vi "Configure Record Parameters (5772).vi"(6 "Record Count":u16=1, 7 "Record Length":u16=3000, 8 "error in":errorcluster, 9 "% of Acquisition Hold Off Time":dbl=10.0, 10 "% of Pre-Trigger Samples":dbl=10.0, 11 "FPGA VI Reference In":refnum<k20>) -> (0 "error out":errorcluster, 3 "FPGA VI Reference Out":refnum<k20>)   [LabVIEW 2012]
uses:
  <vilib>/rvi/errors/niLvFpgaAdjustHostInterfaceError.vi
  <vilib>/rvi/interface/nirviReadWriteControl/nirviReadWriteControl.xnode
  NiFpgaLv.dll
  <vilib>/rvi/interface/Simulation/niFpgaSimulationCallBeginRW.vi
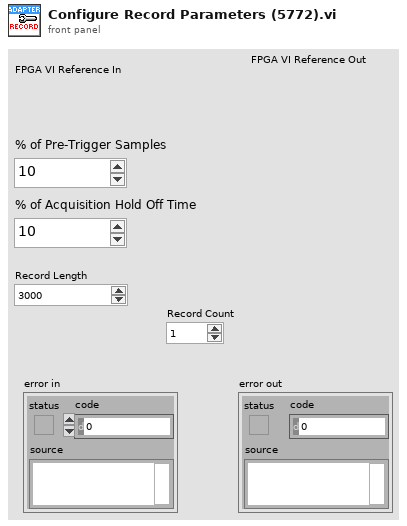
[diagram p1: front panel]
types:
  T1 = cluster{"Load Record Parameters?":bool, "Pre Trigger Samples":u16, "Samples per Record":u16, "Trigger Hold Off":u16, "Record Count":u16}
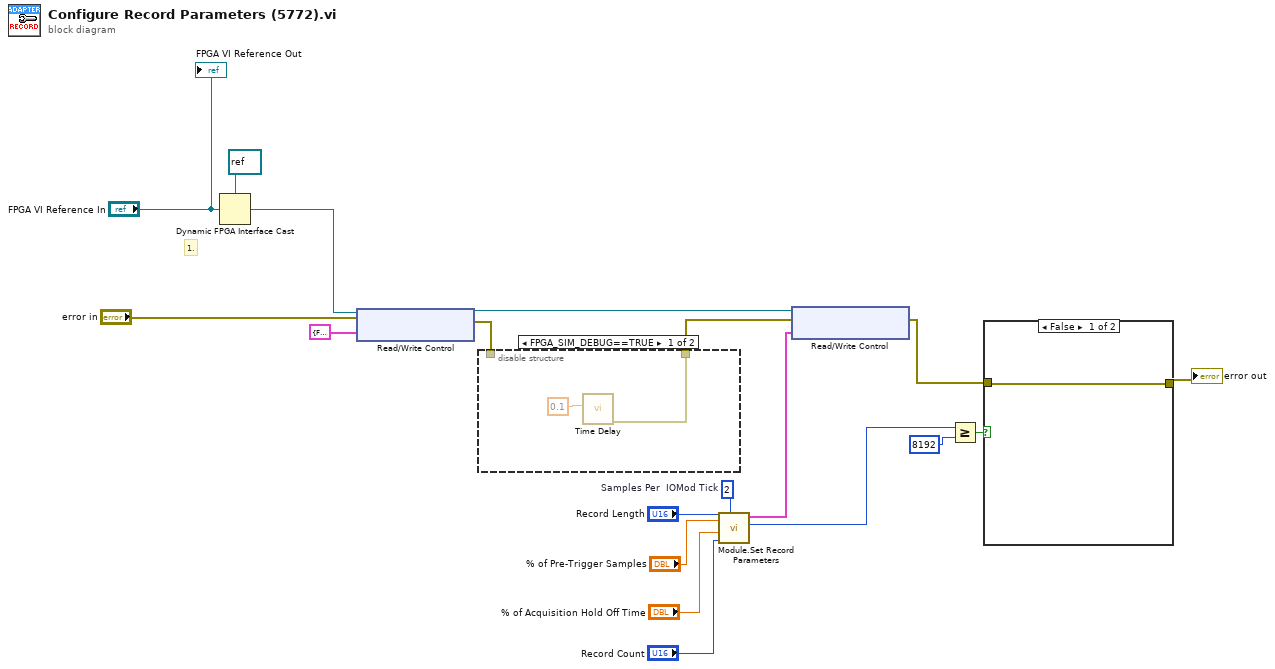
[diagram p0: block diagram]
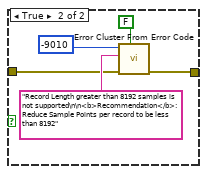
[diagram p3: hidden frame]
diagram:
  w1 = u16 2  # Samples Per  IOMod Tick
  # "1."
  n1 = Dynamic FPGA Interface Cast(Session In=refnum<k20> refnum ("Type"), Type="FPGA VI Reference In") -> (Session Out=w12:refnum<k20>)
  n2 = xnode "Read/Write Control"("FPGA VI Reference In"=w12, "error in"="error in", "Record Parameters"=T1 {"Load Record Parameters?"=FALSE, "Pre Trigger Samples"=0, "Samples per Record"=0, "Trigger Hold Off"=0, "Record Count"=0}) -> ("FPGA VI Reference Out"=w7:refnum<k20>, "error out"=w6:errorcluster)
  n3 = disable-structure shown="FPGA_SIM_DEBUG==TRUE" {
    disable-tunnel: w6 -> [_ w22]
    disable-tunnel: [w20 w22] -> w5
    frame condition #0 {
      n4 = call "Time Delay"("Delay Time (s)"=0.1) -> ("error out"=w20:errorcluster)  [unwired: 10 in]
    }
    frame condition #1 (active) {
    }
  }
  n5 = call <userlib>:"Module.Set Record Parameters.vi"("Samples Per  IOMod Tick"=w1, "Record Count"="Record Count", "% of Hold Off Time"="% of Acquisition Hold Off Time", "% of Pre-Trigger Samples"="% of Pre-Trigger Samples", "Total Number of Samples"="Record Length") -> ("Actual Record Length"=w2:u16, "Record Parameters"=w4:T1)  [unwired: 3 in, 2 out]
  n6 = xnode "Read/Write Control"("FPGA VI Reference In"=w7, "error in"=w5, "Record Parameters"=w4) -> ("error out"=w3:errorcluster)  [unwired: 1 out]
  n7 = Greater Or Equal?(x=w2, y=u16 8192) -> (x >= y?=w8:bool)
  n8 = case shown="False" w8 {
    tunnel: [w23 w28] -> w10
    tunnel: w3 -> [w23 w24]
    frame False {
    }
    frame True {
      n9 = call <vilib>:"Error Cluster From Error Code.vi"("show call chain? (False)"=FALSE, "error in (no error)"=w24, "error message (\"\")"="Record Length greater than 8192 samples is not supported\n\n<b>Recommendation</b>: Reduce Sample Points per record to be less than 8192" ("source"), "error code (0)"=-9010 ("code")) -> ("error out"=w28:errorcluster)  [unwired: 5 in]
    }
  }
  "error out" <- w10
  "FPGA VI Reference Out" <- "FPGA VI Reference In"
